vi "_Drivers Tree.vi"   [LabVIEW 2011]
uses:
  VNA/VNA Command.ctl
  DMM/DMM Command.ctl
  SWI/SWI Command.ctl
  PIM/PIM Command.ctl
  IMP/IMP Command.ctl
  SNA/SNA Command.ctl
  ATT/ATT Command.ctl
  PFE/PFE Command.ctl
  PWM/PWM Command.ctl
panel:
  # "See Diagram"
types:
  T1 = typedef "PWM Command.ctl" = enum16{"LOAD", "INITIALIZE", "PRESET", "GET STIMULUS", "SET STIMULUS", "MEASURE", "RELEASE", "UNLOAD", "GET CALIBRATION", "CALIBRATE"}
  T2 = typedef "PFE Command.ctl" = enum16{"LOAD", "INITIALIZE", "PRESET", "SET STIMULUS", "GET STIMULUS", "GET INFO", "RELEASE", "UNLOAD"}
  T3 = typedef "ATT Command.ctl" = enum16{"LOAD", "INITIALIZE", "PRESET", "SET STIMULUS", "GET STIMULUS", "GET CALIBRATION", "CALIBRATE", "GET INFO", "RELEASE", "UNLOAD"}
  T4 = typedef "SNA Command.ctl" = enum16{"LOAD", "INITIALIZE", "PRESET", "GET STIMULUS", "SET STIMULUS", "GET CALIBRATION", "CALIBRATE", "RESTORE", "MEASURE", "RELEASE", "UNLOAD", "CONFIRM", "SORT"}
  T5 = typedef "IMP Command.ctl" = enum16{"LOAD", "INITIALIZE", "IMPORT", "UNLOAD"}
  T6 = typedef "PIM Command.ctl" = enum16{"LOAD", "KEEP ALIVE", "VALIDATE", "INITIALIZE", "PRESET", "GET CALIBRATION", "SET STIMULUS", "TOGGLE TX POWER", "SET TX ON", "SET TX OFF", "MEASURE", "UNLOAD"}
  T7 = typedef "SWI Command.ctl" = enum16{"LOAD", "INITIALIZE", "PRESET", "SET STIMULUS", "GET STIMULUS", "GET INFO", "RELEASE", "UNLOAD"}
  T8 = typedef "DMM Command.ctl" = enum16{"LOAD", "INITIALIZE", "PRESET", "GET STIMULUS", "SET STIMULUS", "MEASURE", "RELEASE", "UNLOAD", "GET CALIBRATION", "CALIBRATE"}
  T9 = typedef "VNA Command.ctl" = enum16{"LOAD", "INITIALIZE", "PRESET", "GET STIMULUS", "SET STIMULUS", "GET CALIBRATION", "CALIBRATE", "RESTORE", "MEASURE", "RELEASE", "UNLOAD", "CONFIRM", "SORT"}
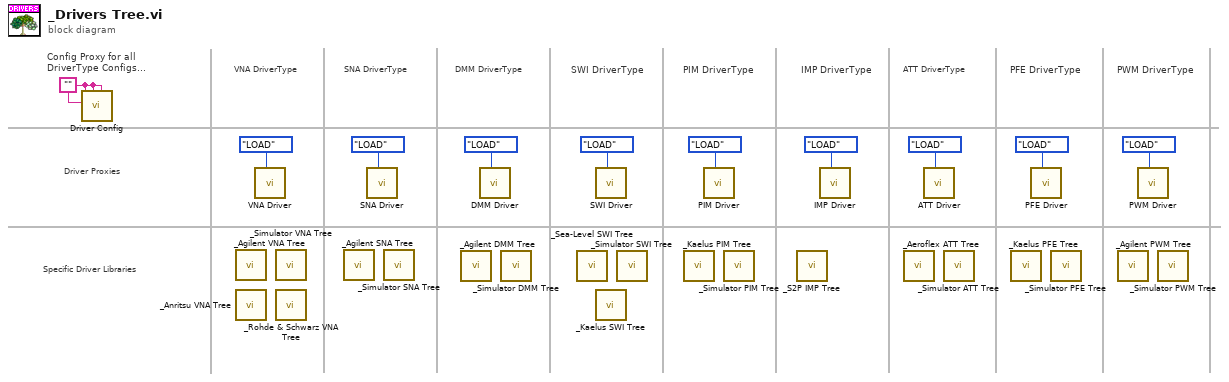
[diagram p0: block diagram]
diagram:
  w5 = ""
  # "PWM DriverType"
  # "PFE DriverType"
  # "ATT DriverType"
  # "SNA DriverType"
  # "IMP DriverType"
  # "PIM DriverType"
  # "SWI DriverType"
  # "DMM DriverType"
  # "Specific Driver Libraries"
  # "Driver Proxies"
  # "VNA DriverType"
  # "Config Proxy for all\nDriverType Configs..."
  n1 = call "Driver Config.vi"("DriverID (\"\")"=w5, "DriverType (\"\")"=w5, "Configuration In (Empty)"=w5, "TestStation Client (\"\")"=w5) -> ()  [unwired: 2 in, 6 out]
  n2 = call "_Agilent VNA Tree.vi"() -> ()  [unwired: 1 out]
  n3 = call "_Anritsu VNA Tree.vi"() -> ()  [unwired: 1 out]
  n4 = call "VNA Driver.vi"("VNA Command"=VNA_Command."LOAD") -> ()  [unwired: 6 in, 5 out]
  n5 = call "_Simulator VNA Tree.vi"() -> ()  [unwired: 1 out]
  n6 = call "_Rohde & Schwarz VNA Tree.vi"() -> ()  [unwired: 1 out]
  n7 = call "_Agilent SNA Tree.vi"() -> ()  [unwired: 1 out]
  n8 = call "SNA Driver.vi"("SNA Command"=SNA_Command."LOAD") -> ()  [unwired: 6 in, 5 out]
  n9 = call "_Simulator SNA Tree.vi"() -> ()  [unwired: 1 in]
  n10 = call "_Agilent DMM Tree.vi"() -> ()  [unwired: 1 out]
  n11 = call "DMM Driver.vi"("DMM Command"=DMM_Command."LOAD" ("VNA Command")) -> ()  [unwired: 4 in, 7 out]
  n12 = call "_Simulator DMM Tree.vi"() -> ()  [unwired: 1 out]
  n13 = call "_Sea-Level SWI Tree.vi"() -> ()  [unwired: 1 out]
  n14 = call "SWI Driver.vi"("SWI Command"=SWI_Command."LOAD") -> ()  [unwired: 4 in, 7 out]
  n15 = call "_Kaelus SWI Tree.vi"() -> ()  [unwired: 1 in]
  n16 = call "_Simulator SWI Tree.vi"() -> ()  [unwired: 1 out]
  n17 = call "_Kaelus PIM Tree.vi"() -> ()  [unwired: 1 out]
  n18 = call "PIM Driver.vi"("PIM Command"=PIM_Command."LOAD") -> ()  [unwired: 4 in, 7 out]
  n19 = call "_Simulator PIM Tree.vi"() -> ()  [unwired: 1 in]
  n20 = call "_S2P IMP Tree.vi"() -> ()  [unwired: 1 out]
  n21 = call "IMP Driver.vi"("IMP Command"=IMP_Command."LOAD" ("VNA Command")) -> ()  [unwired: 4 in, 7 out]
  n22 = call "_Aeroflex ATT Tree.vi"() -> ()  [unwired: 1 in]
  n23 = call "ATT Driver.vi"("ATT Command"=ATT_Command."LOAD") -> ()  [unwired: 7 in, 4 out]
  n24 = call "_Simulator ATT Tree.vi"() -> ()  [unwired: 1 in]
  n25 = call "_Kaelus PFE Tree.vi"() -> ()  [unwired: 1 in]
  n26 = call "PFE Driver.vi"("PFE Command"=PFE_Command."LOAD") -> ()  [unwired: 7 in, 4 out]
  n27 = call "_Simulator PFE Tree.vi"() -> ()  [unwired: 1 in]
  n28 = call "_Agilent PWM Tree.vi"() -> ()  [unwired: 1 in]
  n29 = call "PWM Driver.vi"("PWM Command"=PWM_Command."LOAD") -> ()  [unwired: 7 in, 4 out]
  n30 = call "_Simulator PWM Tree.vi"() -> ()  [unwired: 1 in]
